vi "Check Errors.vi"(8 "Error In":errorcluster, 11 "Central Message Handler In":refnum<class "Central Message Handler.lvclass">) -> (0 "Error Out":errorcluster, 3 "Central Message Handler Out":refnum<class "Central Message Handler.lvclass">)   [LabVIEW 2021, in "Central Message Handler.lvclass"]
uses:
  Central Message Handler.lvclass
  Process/Public/Controls/Process Message.ctl
  Process/Process.lvclass
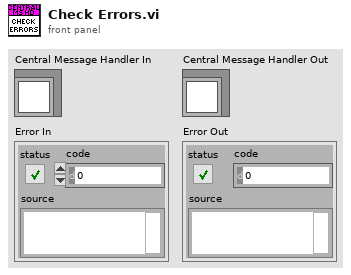
[diagram p1: front panel]
types:
  T1 = typedef "Process.lvclass/Process Message.ctl" = cluster{"Command":string, "Data":variant}
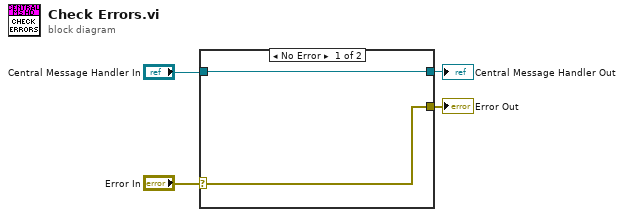
[diagram p0: block diagram]
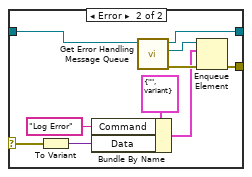
[diagram p2: hidden frame]
diagram:
  n1 = case shown="No Error" "Error In" {
    selector: "Error In" -> [w5 w15]
    tunnel: [w5 w13] -> w1
    tunnel: "Central Message Handler In" -> [w6 w12]
    tunnel: [w6 w11] -> w2
    frame No Error {
    }
    frame Error {
      n2 = To Variant(anything=w15) -> (Variant=w16:variant)
      n3 = Bundle By Name(cluster=T1 {"Command"="", "Data"=variant} ("element"), "Command"="Log Error", "Data"=w16) -> (w7:T1)
      n4 = call "Get Error Handling Message Queue.vi"("Central Message Handler In"=w12) -> ("Error Out"=w9:errorcluster, "Error Handling Message Queue"=w10:refnum<queue>, "Central Message Handler Out"=w11:refnum<class "Central Message Handler.lvclass">)  [unwired: 8 in]
      n5 = Enqueue Element(queue=w10, element=w7, error in (no error)=w9) -> (error out=w13:errorcluster)  [unwired: 1 in, 2 out]
    }
  }
  "Central Message Handler Out" <- w2
  "Error Out" <- w1
